vi "PS Channel UI.vi"() -> ()   [LabVIEW 2025, in "Power Supply.lvlib" / "Power Supply Channel.lvclass"]
doc: "Copyright 2017 National Instruments Corporation\n\nLicensed under the Apache License, Version 2.0 (the \"License\"); you may not use this file except in compliance with the License. You may obtain a copy of the License at http://www.apache.org/licenses/LICENSE-2.0\nUnless required by applicable law or agreed to in writing, software distributed under the License is distributed on an \"AS IS\" BASIS, WITHOUT WARRANTIES OR CONDITIONS OF ANY KIND, either express or implied. See the License for the specific language governing permissions and limitations under the License."
uses:
  Power Supply Channel.lvclass
  Users/Public/Documents/Sandia National Labs/TSS Plugin/CEF.lvlibp/Node/NodeRef.ctl
  Users/Public/Documents/Sandia National Labs/TSS Plugin/CEF.lvlibp/Node/CEF_Node.lvclass
  Users/Public/Documents/Sandia National Labs/TSS Plugin/CEF.lvlibp/Node/mainQref.ctl
  Users/Public/Documents/Sandia National Labs/TSS Plugin/CEF.lvlibp/Node/UserEventRef.ctl
  Users/Public/Documents/Sandia National Labs/TSS Plugin/Abstract Engine.lvlibp/Channel configuration/Default Channel.ctl
  PS Channel configuration/PS Channel Setting.ctl
  C:/Users/Public/Documents/Sandia National Labs/TSS Plugin/CEF.lvlibp/Node/CEF_Node.lvclass
  Power Supply Channel.lvclass/Power Supply Channel.ctl
  PS Channel configuration/Power Supply Channel configuration.lvclass/Power Supply Channel configuration.ctl
  PS Channel configuration/Read PS Channel.vi
  PS Channel configuration/Write PS Channel.vi
  <vilib>/Utility/error.llb/Trim Whitespace One-Sided.vi
  PS Channel configuration/Power Supply Channel configuration.lvclass
  C:/Users/Public/Documents/Sandia National Labs/TSS Plugin/Abstract Engine.lvlibp/Channel configuration/Channel configuration.lvclass
  Users/Public/Documents/Sandia National Labs/TSS Plugin/Abstract Engine.lvlibp/Channel configuration/Read Channel Setting.vi
  Users/Public/Documents/Sandia National Labs/TSS Plugin/Abstract Engine.lvlibp/Channel configuration/Write Channel Setting.vi
  Users/Public/Documents/Sandia National Labs/TSS Plugin/Abstract Engine.lvlibp/Channel configuration/Channel configuration.lvclass
panel:
  in  "PS Channel":cluster{"Default":T1, "Setting":T2}={"Default"={"Address"="None", "SW Alias"="", "Enabled"=TRUE, "Type"="", "Description"="* Channel Type = Channel Class"}, "Setting"={"Driver"="", "Pin"="", "Test Voltage"="", "Voltage Low"=1.0, "Voltage Norminal"=1.0, "Voltage High"=1.0, "PreTest Voltage"=0.0, "PreTest Current"=0.0, "Current Limit"=0.1}}
  in  "user event":T3
  in  "main queue":T4
  in  "node ref":T5
  # "Output Control"
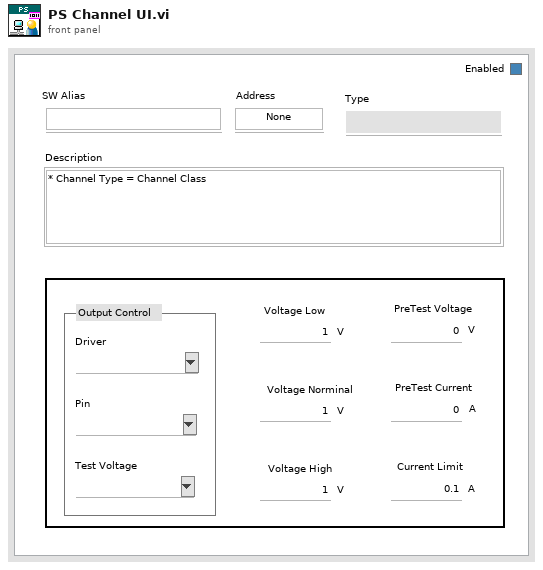
[diagram p1: front panel]
types:
  T1 = typedef "Abstract Engine.lvlibp/Channel configuration.lvclass/Default Channel.ctl" = cluster{"Address":string, "SW Alias":string, "Enabled":bool, "Type":string, "Description":string}
  T2 = typedef "Power Supply.lvlib/Power Supply Channel configuration.lvclass/PS Channel Setting.ctl" = cluster{"Driver":string, "Pin":string, "Test Voltage":string, "Voltage Low":dbl, "Voltage Norminal":dbl, "Voltage High":dbl, "PreTest Voltage":dbl, "PreTest Current":dbl, "Current Limit":dbl}
  T3 = typedef "CEF.lvlibp/CEF_Node.lvclass/UserEventRef.ctl" = refnum<user-event>
  T4 = typedef "CEF.lvlibp/CEF_Node.lvclass/mainQref.ctl" = refnum<queue>
  T5 = typedef "CEF.lvlibp/CEF_Node.lvclass/NodeRef.ctl" = refnum<data-value>
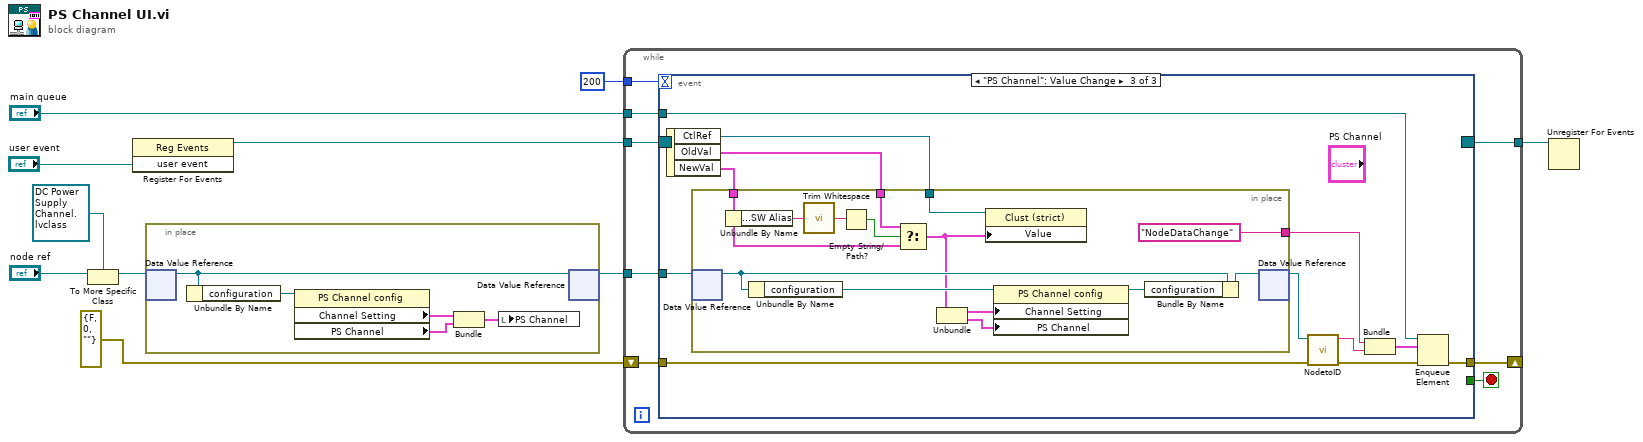
[diagram p0: block diagram]
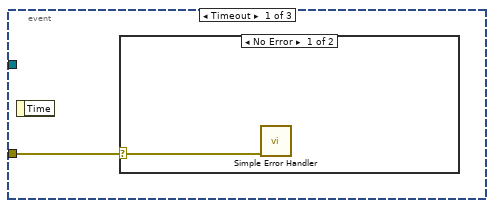
[diagram p2: hidden frame]
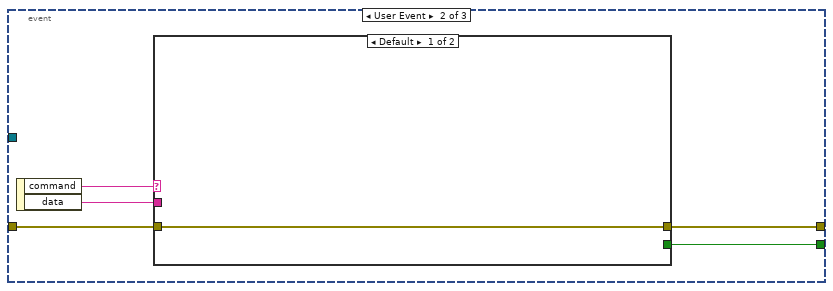
[diagram p4: hidden frame]
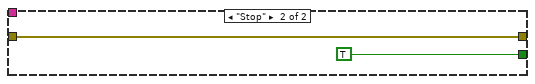
[diagram p5: hidden frame]
diagram:
  n1 = To More Specific Class(target class=refnum<data-value> refnum ("data value reference"), reference="node ref") -> (specific class reference=w4:refnum<data-value>)  [unwired: 1 in, 1 out]
  n2 = register-events("user event") -> (reference out=w9:refnum<event-registration>)  [unwired: 2 in, 1 out]
  n3 = in-place {
    # "Initialize the front panel controls when loaded"
    n4 = in-place-dvr #1(w4) -> (w15:refnum<class "Power Supply Channel.lvclass">)  [unwired: 1 out]
    n5 = Unbundle By Name(w15) -> ("configuration"=w14:refnum<class "Power Supply Channel configuration.lvclass">)
    n6 = property class="PS Channel config"(reference=w14) -> ("Channel Setting"=w13:T1, "PS Channel"=w12:T2)  [unwired: 1 in, 2 out]
    n7 = Bundle("Channel Setting"=w13, "PS Channel"=w12) -> (w11:cluster{"Channel Setting":T1, "PS Channel":T2})  [unwired: 1 in]
    n8 = local write "PS Channel"(w11) -> ()
    n9 = in-place-dvr #1(w15) -> (w3:refnum<data-value>)  [unwired: 1 out]
  }
  n10 = while {
    tunnel: w3 -> [w23]
    tunnel: w9 -> [w22]
    tunnel: [w21] -> w8
    tunnel: "main queue" -> [w18]
    tunnel: 200 -> [w16]
    shift-right: [w19] -> _
    shift-left: errorcluster {"status"=FALSE, "code"=0, "source"=""} ("error out") -> [w17]
    stop <- w20 stop-if-true
    n11 = event shown="[2] \"PS Channel\": Value Change" {
      selector: w22 -> [_ _ _]
      dyn-events: [_ _ _] -> w21
      timeout: w16 -> [_ _ _]
      tunnel: w23 -> [_ _ w43]
      tunnel: [_ w28 _] -> w20
      tunnel: [_ w26 w44] -> w19
      tunnel: w18 -> [_ _ w45]
      tunnel: w17 -> [w24 w27 w35]
      event Timeout {
        n12 = event-data() -> ()  [unwired: 1 in, 1 out]
        n13 = case shown="No Error" w24 {
          selector: w24 -> [w25 _]
          frame No Error {
            n14 = call <vilib>:"Simple Error Handler.vi"("error in (no error)"=w25) -> ()  [unwired: 4 in, 5 out]
          }
          frame Error {
          }
        }
      }
      event User Event {
        n15 = event-data() -> ("command"=w30:string, "data"=w29:string)  [unwired: 1 in]
        n16 = case shown="Default" w30 {
          tunnel: w29 -> [_ _]
          tunnel: [_ TRUE] -> w28
          tunnel: w27 -> [w31 w32]
          tunnel: [w31 w32] -> w26
          frame Default {
          }
          frame "Stop" {
          }
        }
      }
      event "PS Channel": Value Change {
        n17 = event-data() -> ("CtlRef"=w39:refnum<vi>, "OldVal"=w41:cluster{"Default":T1, "Setting":T2}, "NewVal"=w40:cluster{"Default":T1, "Setting":T2})  [unwired: 1 in]
        n18 = in-place {
          in-place-border: w41 -> [w55]
          in-place-border: w40 -> [w52]
          in-place-border: w39 -> [w54]
          in-place-border: ["NodeDataChange" ("Message Name")] -> w38
          n19 = in-place-dvr #2(w43) -> (w59:refnum<class "Power Supply Channel.lvclass">)  [unwired: 1 out]
          n20 = Unbundle By Name(w52) -> ("Default.SW Alias"=w53:string)
          n21 = Unbundle By Name(w59) -> ("configuration"=w58:refnum<class "Power Supply Channel configuration.lvclass">)
          n22 = call <vilib>:"Trim Whitespace.vi"("string"=w53) -> ("trimmed string"=w50:string)  [unwired: 1 in]
          n23 = Empty String/Path?(string/path=w50) -> (empty?=w51:bool)
          n24 = Select(t=w55, s=w51, f=w52) -> (s? t:f=w49:cluster{"Default":T1, "Setting":T2})
          n25 = Unbundle(w49) -> ("Default"=w46:T1, "Setting"=w48:T2)
          n26 = property class="Clust (strict)"(reference=w54, "Value"=w49) -> ()  [unwired: 1 in, 2 out]
          n27 = property class="PS Channel config"(reference=w58, "Channel Setting"=w46, "PS Channel"=w48) -> (reference out=w56:refnum<class "Power Supply Channel configuration.lvclass">)  [unwired: 1 in, 1 out]
          n28 = Bundle By Name(cluster=w59, "configuration"=w56) -> (w57:refnum<class "Power Supply Channel.lvclass">)
          n29 = in-place-dvr #2(w57) -> (w42:refnum<data-value>)  [unwired: 1 out]
        }
        n30 = call "NodetoID.vi"("error in"=w35, "node ref"=w42) -> ("error out"=w34:errorcluster, "ID"=w37:string)  [unwired: 8 in]
        n31 = Bundle("Message Name"=w38, "ID"=w37) -> (w36:cluster{"Message Name":string, "ID":string})  [unwired: 1 in]
        n32 = Enqueue Element(queue=w45, element=w36, error in (no error)=w34) -> (error out=w44:errorcluster)  [unwired: 1 in, 2 out]
      }
    }
  }
  n33 = Unregister For Events(event registration refnum=w8) -> ()  [unwired: 1 in, 1 out]
